vi "Cluster to Array (recursive).vi"(8 "error in (no error)":errorcluster, 11 "Variant":variant) -> (0 "error out":errorcluster, 2 "Elements":variant[](array[variant]), 3 "Types":T1[](array[typedef]))   [LabVIEW 2016, in "PQ Connection.lvclass"]
uses:
  PQ Connection.lvclass
  <vilib>/Utility/Data Type/NI_Data Type.lvlib
  <vilib>/Utility/Data Type/Type Definitions/Data Type.ctl
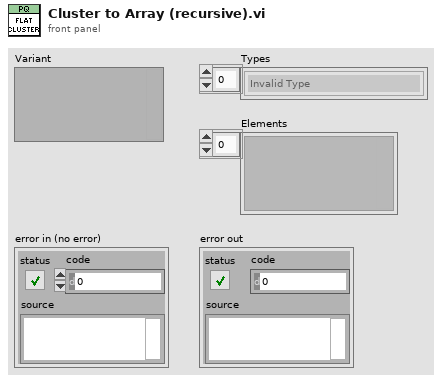
[diagram p1: front panel]
types:
  T1 = typedef "NI_Data Type.lvlib/Data Type.ctl" = enum8{"Invalid Type", "Void", "I8", "I16", "I32", "I64", "U8", "U16", "U32", "U64", "Single Float", "Double Float", "Extended Float", "Single Complex", "Double Complex", "Extended Complex", "Enum U8", "Enum U16", "Enum U32", "Enum U64", "Single Float With Unit", "Double Float With Unit", "Extended Float With Unit", "Single Complex with Unit", "Double Complex with Unit", "Extended Complex with Unit", "Boolean", "String", "Path", "Picture", "Tag", "Array", "Cluster", "Variant", "LV Variant", "Waveform", "Timestamp", "Digital Waveform", "Digital Data", "ExpressData", "Refnum", "External Data", "VI", "Poly VI", "LabVIEW Class Instance", "Fixed Point", "Set Collection", "Map Collection"}
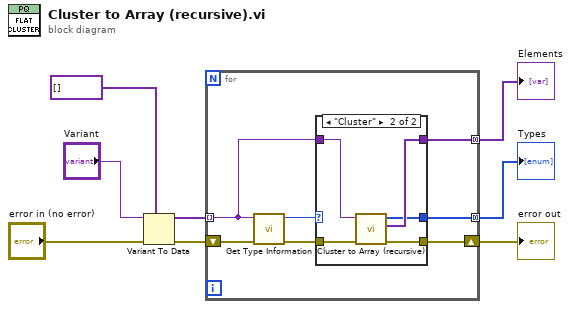
[diagram p0: block diagram]
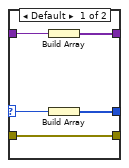
[diagram p2: hidden frame]
diagram:
  n1 = Variant To Data(error in="error in (no error)", type=variant[] [], Variant="Variant") -> (data=w6:variant[], error out=w2:errorcluster)
  n2 = for {
    tunnel: w6 -> [w15] mode=indexing
    tunnel: [w14] -> w7 mode=concatenating
    tunnel: [w12] -> w8 mode=concatenating
    shift-right: [w9] -> w1
    shift-left: w2 -> [w11]
    n3 = call <vilib>:"Get Type Information.vi"("error in (no error)"=w11, "variant"=w15) -> ("error out"=w10:errorcluster, "type"=w13:T1)  [unwired: 5 in, 3 out]
    n4 = case shown="\"Cluster\"" w13 {
      selector: w13 -> [w18 _]
      tunnel: w15 -> [w20 w25]
      tunnel: [w19 w24] -> w14
      tunnel: [w17 w23] -> w12
      tunnel: w10 -> [w16 w22]
      tunnel: [w16 w21] -> w9
      frame Default {
        n5 = Build Array(w20) -> (w19:variant[])
        n6 = Build Array(w18) -> (w17:T1[])
      }
      frame "Cluster" {
        n7 = call "Cluster to Array (recursive).vi"("error in (no error)"=w22, "Variant"=w25) -> ("error out"=w21:errorcluster, "Elements"=w24:variant[], "Types"=w23:T1[])  [unwired: 7 in]
      }
    }
  }
  "Types" <- w8
  "Elements" <- w7
  "error out" <- w1
